vi "test_decodeMonEntry.vi"() -> ()   [LabVIEW 2020]
uses:
  <instrlib>/AIM GmbH/_AIM 664/helpers/EthFrameManagement/controls/ehternetFrame_type.ctl
  <instrlib>/AIM GmbH/_AIM 664/helpers/EthFrameManagement/controls/IPFrame_type.ctl
  <instrlib>/AIM GmbH/_AIM 664/helpers/EthFrameManagement/controls/UDPFrame_type.ctl
  <instrlib>/AIM GmbH/_AIM 664/_controls/monitor_fhInfol_type.ctl
  <instrlib>/AIM GmbH/_AIM 664/_controls/monitor_entrySize_type.ctl
  <instrlib>/AIM GmbH/_AIM 664/_controls/monitor_fhw0_type.ctl
  <instrlib>/AIM GmbH/_AIM 664/_controls/monitor_fhw1_type.ctl
  <instrlib>/AIM GmbH/_AIM 664/_controls/monitor_becw_type.ctl
  <instrlib>/AIM GmbH/_AIM 664/helpers/EthFrameManagement/EthFrameManagement.lvlib
  <instrlib>/AIM GmbH/_AIM 664/AIM664LV.lvlib
panel:
  in  "ReadBuffer":u8[](array[numeric]) format="%.0x"
  out "FwIrigTime":cluster{"TtHigh":u32, "TtLow":u32}
  out "BECW":T1
  out "FrameHeaderInfo":T2 {"FHW0"."MacID" format="%03b"}
  in  "header size bytes (32)":i32=32
  out "dst ip":string
  out "src ip":string
  out "size(s)":i32
  out "UDP header":T6
  out "IP header":T7 {"CtlFlags" format="%.0b"; "Dest IP" format="%.0x"; "Source IP" format="%.0x"; "Checksum" format="%.0x"; "TTL" format="%.0x"; "FragOffset" format="%.0x"; "ID" format="%.0x"; "Length" format="%.0x"; "ToS" format="%.0x"; "IHL" format="%.0x"; "Version" format="%.0x"}
  out "UDP Header Only":u8[](array[numeric])
  out "IP Header Only":u8[](array[numeric]) format="%.0x"
  out "Ethernet header":T8 {"EtherType" format="%04x"; "Src MAC" format="%02x"; "Dest MAC" format="%.0x"}
  out "MAC Header Only":u8[](array[numeric]) format="%.0x"
  out "payload":u8[](array[numeric]) format="%.0x"
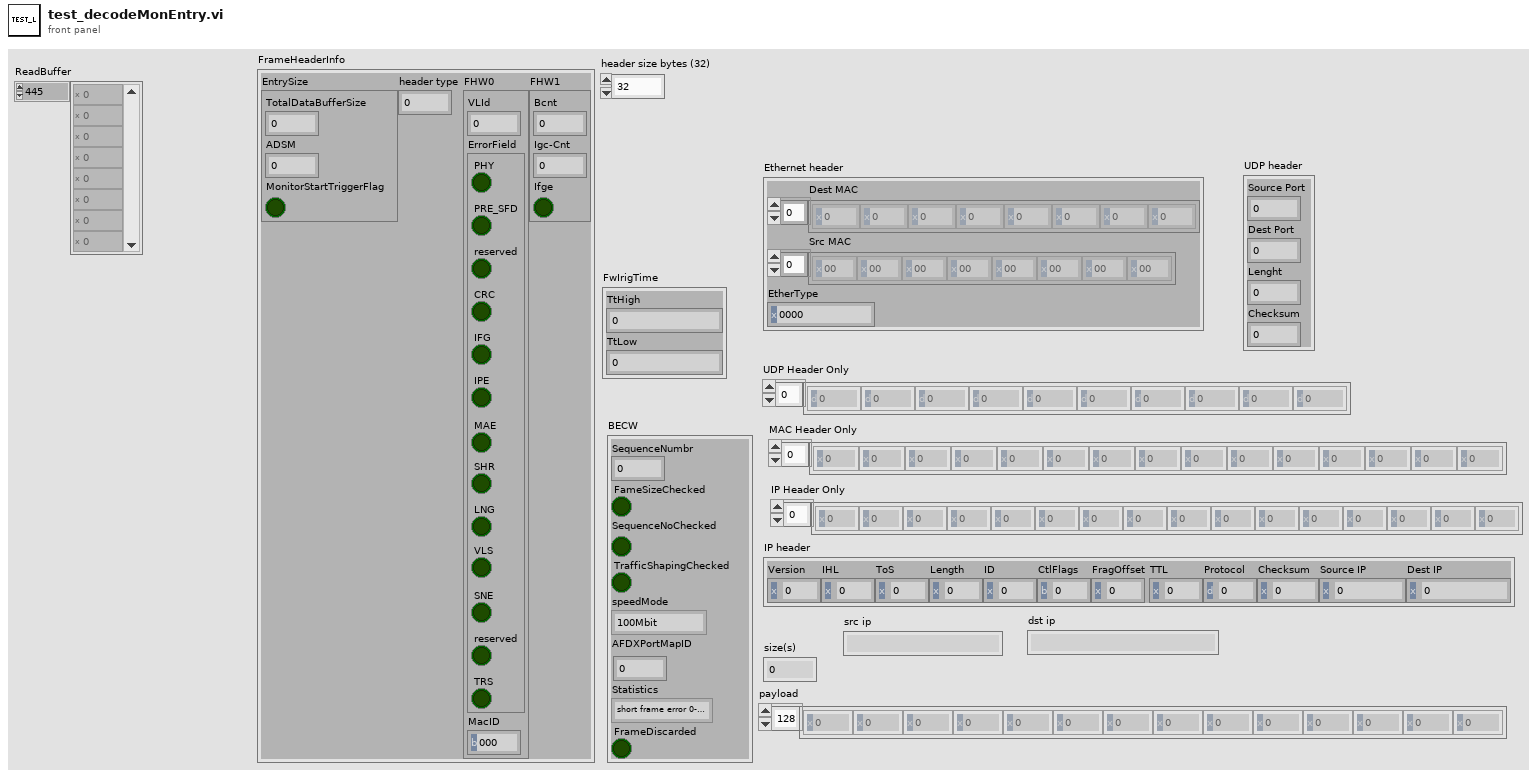
[diagram p1: front panel]
types:
  T1 = typedef "AIM664LV.lvlib/monitor_becw_type.ctl" = cluster{"SequenceNumbr":u8, "FameSizeChecked":bool, "SequenceNoChecked":bool, "TrafficShapingChecked":bool, "speedMode":enum16{"100Mbit", "10Mbit", "1Gbit"}, "AFDXPortMapID":u8, "Statistics":enum16{"short frame error 0-63Bytes", "64-127 Bytes", "128-255 Bytes", "256-511 Bytes", "512-1023 Bytes", "1024-1518 Bytes", ">1518 Bytes"}, "FrameDiscarded":bool}
  T2 = typedef "AIM664LV.lvlib/monitor_fhInfol_type.ctl" = cluster{"EntrySize":T3, "header type":u32, "FHW0":T4, "FHW1":T5}
  T3 = typedef "AIM664LV.lvlib/monitor_entrySize_type.ctl" = cluster{"TotalDataBufferSize":u16, "ADSM":u16, "MonitorStartTriggerFlag":bool}
  T4 = typedef "AIM664LV.lvlib/monitor_fhw0_type.ctl" = cluster{"VLId":u16, "ErrorField":cluster{"PHY":bool, "PRE_SFD":bool, "reserved":bool, "CRC":bool, "IFG":bool, "IPE":bool, "MAE":bool, "SHR":bool, "LNG":bool, "VLS":bool, "SNE":bool, "reserved":bool, "TRS":bool}, "MacID":u8}
  T5 = typedef "AIM664LV.lvlib/monitor_fhw1_type.ctl" = cluster{"Bcnt":u16, "Igc-Cnt":u16, "Ifge":bool}
  T6 = typedef "EthFrameManagement.lvlib/UDPFrame_type.ctl" = cluster{"Source Port":u16, "Dest Port":u16, "Lenght":u16, "Checksum":u16}
  T7 = typedef "EthFrameManagement.lvlib/IPFrame_type.ctl" = cluster{"Version":u8, "IHL":u8, "ToS":u8, "Length":u16, "ID":u16, "CtlFlags":u8, "FragOffset":u16, "TTL":u8, "Protocol":u8, "Checksum":u16, "Source IP":u32, "Dest IP":u32}
  T8 = typedef "EthFrameManagement.lvlib/ehternetFrame_type.ctl" = cluster{"Dest MAC":u8[], "Src MAC":u8[], "EtherType":u16}
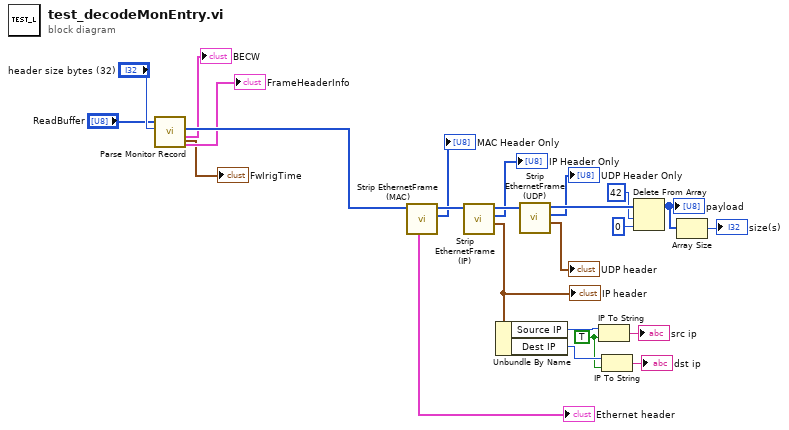
[diagram p0: block diagram]
diagram:
  w9 = TRUE ("dot notation? (F)")
  n1 = call <instrlib>:"Parse Monitor Record.vi"("header size bytes (32)"="header size bytes (32)", "Record In"="ReadBuffer") -> ("FrameHeaderInfo"=→"FrameHeaderInfo":T2, "BECW"=→"BECW":T1, "Payload"=w6:u8[], "FwIrigTime"=→"FwIrigTime":cluster{"TtHigh":u32, "TtLow":u32})  [unwired: 4 in, 2 out]
  n2 = call <instrlib>:"Strip EthernetFrame (MAC).vi"("Ethernet Frame In"=w6) -> ("Ethernet header"=→"Ethernet header":T8, "MAC Header Only"=→"MAC Header Only":u8[], "Ethernet Frame Out"=w24:u8[])  [unwired: 7 in, 1 out]
  n3 = call <instrlib>:"Strip EthernetFrame (IP).vi"("Frame In"=w24) -> ("IP header"=w12:T7, "IP Header Only"=→"IP Header Only":u8[], "Frame Out"=w23:u8[])  [unwired: 7 in, 1 out]
  "IP header" <- w12
  n4 = Unbundle By Name(w12) -> ("Source IP"=w11:u32, "Dest IP"=w10:u32)
  n5 = call <instrlib>:"Strip EthernetFrame (UDP).vi"("Ethernet Frame In"=w23) -> ("UDP header"=→"UDP header":T6, "UDP Header Only"=→"UDP Header Only":u8[], "Ethernet Frame Out"=w22:u8[])  [unwired: 7 in, 1 out]
  n6 = IP To String(1:w9, 2:w11) -> (0:→"src ip":string)
  n7 = IP To String(1:w9, 2:w10) -> (0:→"dst ip":string)
  n8 = Delete From Array(array=w22, length=42 ("index"), index=0) -> (array with subset deleted=w14:u8[])  [unwired: 1 out]
  "payload" <- w14
  n9 = Array Size(array=w14) -> (size(s)=→"size(s)":i32)
